vi "Manipulator Get XYZ.vi"(8 "error in (no error)":errorcluster, 11 "VISA resource in":refnum<visa-resource-name>="COM1") -> (0 "error out":errorcluster, 2 "Coordinates":cluster{"X":i32, "Y":i32, "Z":i32}, 3 "VISA resource out":refnum<visa-resource-name>)   [LabVIEW 2012, in "Scientifica Manipulator Daemon.lvlib"]
uses:
  Scientifica Manipulator Daemon.lvlib
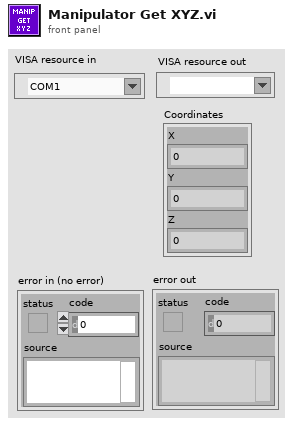
[diagram p1: front panel]
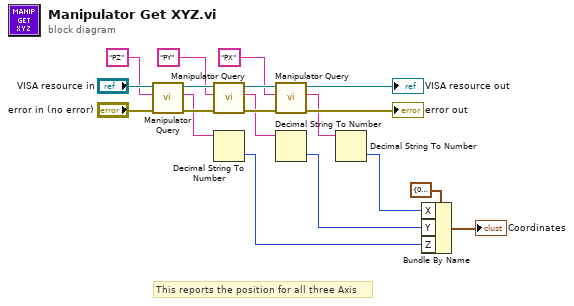
[diagram p0: block diagram]
diagram:
  # "This reports the position for all three Axis"
  n1 = call "Manipulator Query.vi"("error in (no error)"="error in (no error)", "Command"="PZ", "VISA resource in"="VISA resource in") -> ("error out"=w12:errorcluster, "Response"=w4:string, "VISA resource out"=w13:refnum<visa-resource-name>)  [unwired: 5 in, 1 out]
  n2 = call "Manipulator Query.vi"("error in (no error)"=w12, "Command"="PY", "VISA resource in"=w13) -> ("error out"=w10:errorcluster, "Response"=w3:string, "VISA resource out"=w11:refnum<visa-resource-name>)  [unwired: 5 in, 1 out]
  n3 = Decimal String To Number(string=w4) -> (number=w16:i32)  [unwired: 2 in, 1 out]
  n4 = call "Manipulator Query.vi"("error in (no error)"=w10, "Command"="PX", "VISA resource in"=w11) -> ("error out"=→"error out":errorcluster, "Response"=w2:string, "VISA resource out"=→"VISA resource out":refnum<visa-resource-name>)  [unwired: 5 in, 1 out]
  n5 = Decimal String To Number(string=w3) -> (number=w17:i32)  [unwired: 2 in, 1 out]
  n6 = Decimal String To Number(string=w2) -> (number=w18:i32)  [unwired: 2 in, 1 out]
  n7 = Bundle By Name(cluster=cluster{"X":i32, "Y":i32, "Z":i32} {"X"=0, "Y"=0, "Z"=0} ("Dummy Cluster"), "X"=w18, "Y"=w17, "Z"=w16) -> (→"Coordinates":cluster{"X":i32, "Y":i32, "Z":i32})
